vi "CANAnalData.vi"(8 "error in":errorcluster, 9 "ID":u32, 10 "Data":u8[](array[numeric]), 11 "Config":refnum<vi>) -> (0 "error out":errorcluster, 1 "DataLen":u8, 2 "Data out":u8[](array[numeric]), 3 "ID out":u32, 5 "TimeStamp":u32)   [LabVIEW 2017]
uses:
  PCAN_Driver/ControlCAN.llb/VCI_CAN_OBJ.ctl
  Marvin ATP Remake 6.5.18 - Copy/PCAN_Driver/ControlCAN.lvlib
panel:
  in  "cnd_in":u32
  out "cnt_out":u32
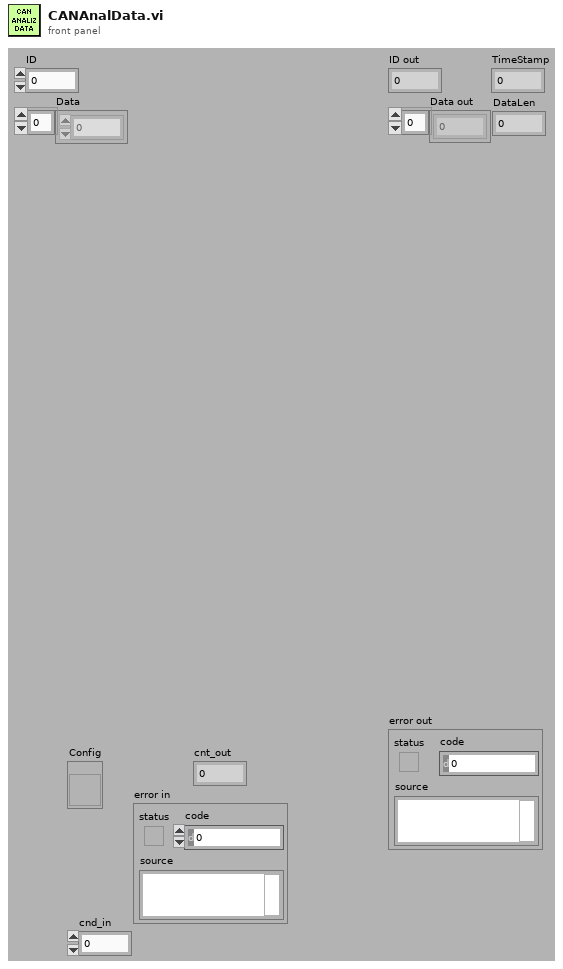
[diagram p1: front panel]
types:
  T1 = typedef "ControlCAN.lvlib/VCI_CAN_OBJ.ctl" = cluster{"ID":u32, "TimeStamp":u32, "TimeFlag":u8, "SendType":u8, "RemoteFlag":u8, "ExternFlag":u8, "DataLen":u8, "Data":u8[], "Reserved":u8[]}
  T2 = typedef "ControlCAN.lvlib/DevType.ctl" = u32
  T3 = typedef "ControlCAN.lvlib/CAN Channel.ctl" = u32
  T4 = typedef "ControlCAN.lvlib/VCI_INIT_CONFIG.ctl" = cluster{"AccCode":u32, "AccMask":u32, "InitFlag":T5, "Fliter":T6, "Timing0":u8, "Timing1":u8, "Mode":T7}
  T5 = typedef "ControlCAN.lvlib/InitFlag.ctl" = u32
  T6 = typedef "ControlCAN.lvlib/Fliter.ctl" = u8
  T7 = typedef "ControlCAN.lvlib/Mode.ctl" = u8
  T8 = cluster{"DevType":T2, "DevIndex":u32, "CanIndex":T3, "VCI_INIT_CONFIG":T4}
  T9 = cluster{"Type":enum16{"接收", "发送"}, "Channel":T3, "Time":timestamp, "VCI_CAN_OBJ":T1}[]
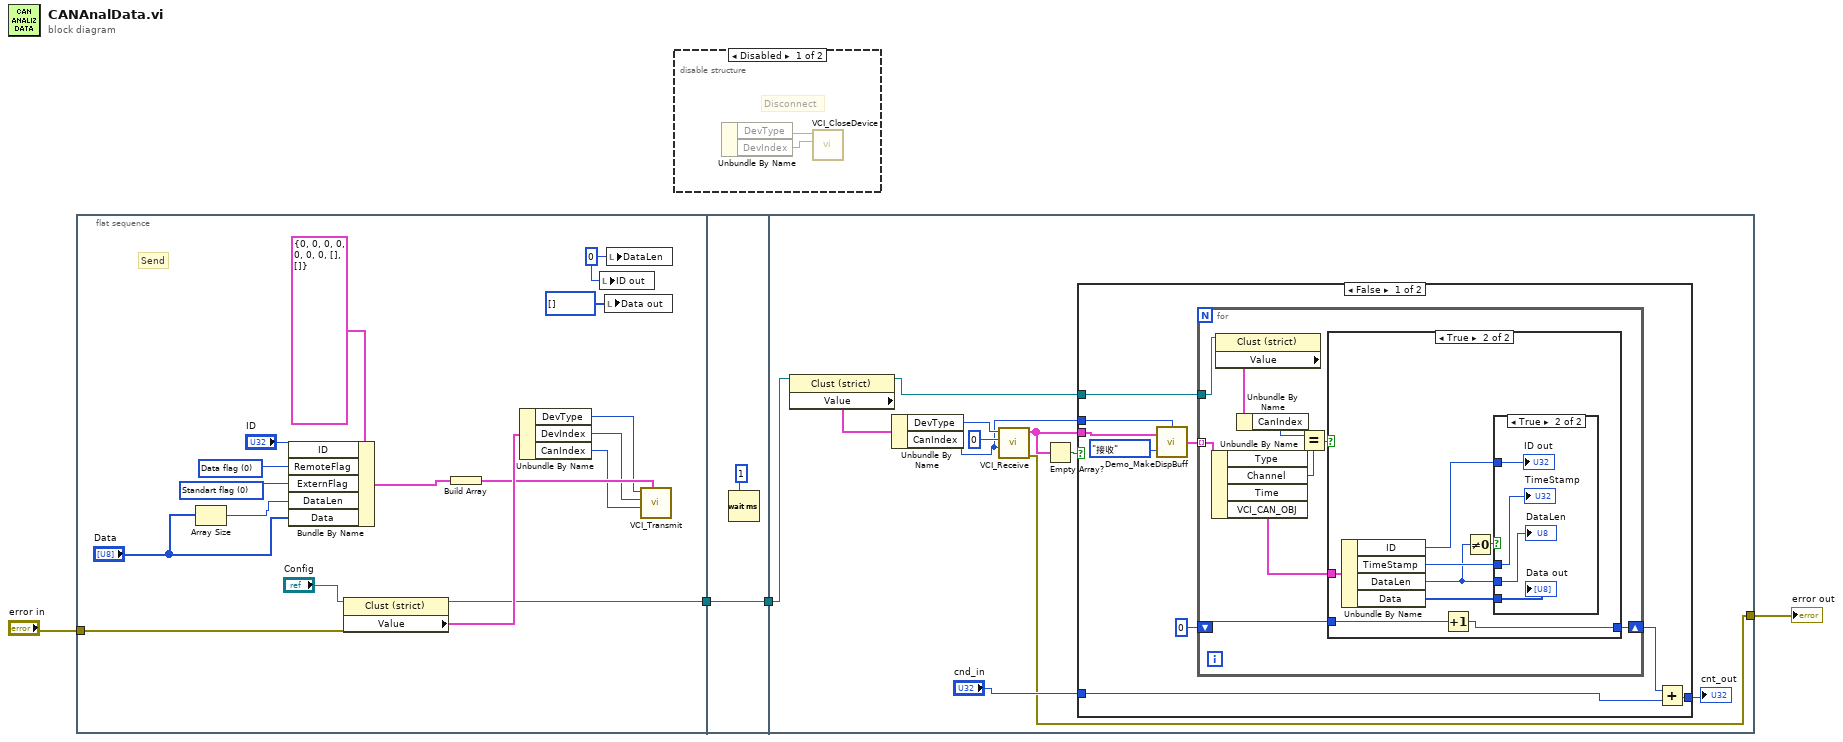
[diagram p0: block diagram]
diagram:
  n1 = flat-sequence {
    tunnel: [w8] -> w4
    tunnel: "error in" -> [w5]
    tunnel: w4 -> [w23]
    tunnel: [w23] -> w3
    tunnel: w3 -> [w25]
    tunnel: [w24] -> w1
    frame #0 {
      w7 = u8 0 ("DataLen")
      w15 = u8 0 items=["Standart flag", "Extern flag"] ("Format")
      w14 = u8 0 items=["Data flag", "Remote flag"] ("Type")
      # "Send"
      n2 = Array Size(array="Data") -> (size(s)=w10:i32)
      n3 = Bundle By Name(cluster=T1 {"ID"=0, "TimeStamp"=0, "TimeFlag"=0, "SendType"=0, "RemoteFlag"=0, "ExternFlag"=0, "DataLen"=0, "Data"=[], "Reserved"=[]} ("Send"), "ID"="ID", "RemoteFlag"=w14, "ExternFlag"=w15, "DataLen"=w10, "Data"="Data") -> (w13:T1)
      n4 = property class="Clust (strict)"(reference="Config", error in=w5) -> (reference out=w8:refnum<vi>, "Value"=w21:T8)  [unwired: 1 out]
      n5 = Build Array(w13) -> (w20:T1[])
      n6 = Unbundle By Name(w21) -> ("DevType"=w17:T2, "DevIndex"=w18:u32, "CanIndex"=w19:T3)
      n7 = local write "ID out"(w7) -> ()
      n8 = local write "Data out"(u8[] [] ("Data out")) -> ()
      n9 = local write "DataLen"(w7) -> ()
      n10 = call "VCI_Transmit.vi"("Buffer"=w20, "CANIndex"=w19, "DevIndex"=w18, "DevType"=w17) -> ()  [unwired: 1 in, 7 out]
    }
    frame #1 {
      n11 = Wait (ms)(milliseconds to wait=u32 1) -> ()  [unwired: 1 out]
    }
    frame #2 {
      n12 = property class="Clust (strict)"(reference=w25) -> (reference out=w34:refnum<vi>, "Value"=w28:T8)  [unwired: 1 in, 1 out]
      n13 = Unbundle By Name(w28) -> ("DevType"=w30:T2, "CanIndex"=w29:T3)
      n14 = call "VCI_Receive.vi"("CANIndex"=w29, "DevIndex"=u32 0, "DevType"=w30) -> ("error out"=w24:errorcluster, "Recieve"=w31:T1[])  [unwired: 3 in, 4 out]
      n15 = Empty Array?(array=w31) -> (empty?=w32:bool)
      n16 = case shown="False" w32 {
        tunnel: w31 -> [w41 _]
        tunnel: w29 -> [w42 _]
        tunnel: "cnd_in" -> [w37 w66]
        tunnel: [w36 w66] -> w27
        tunnel: w34 -> [w35 _]
        frame False {
          n17 = call "Demo_MakeDispBuff.vi"("Channel"=w42, "Type"=enum16{"接收", "发送"}."接收", "OBJs"=w41) -> ("Buffer"=w40:T9)
          n18 = for {
            tunnel: w40 -> [w52] mode=indexing
            shift-right: [w45] -> w38
            shift-left: u32 0 -> [w46]
            tunnel: w35 -> [w44]
            n19 = Unbundle By Name(w52) -> ("Channel"=w48:T3, "VCI_CAN_OBJ"=w51:T1)  [unwired: 2 out]
            n20 = property class="Clust (strict)"(reference=w44) -> ("Value"=w50:T8)  [unwired: 1 in, 2 out]
            n21 = Unbundle By Name(w50) -> ("CanIndex"=w49:T3)
            n22 = Equal?(x=w49, y=w48) -> (x = y?=w47:bool)
            n23 = case shown="True" w47 {
              tunnel: w51 -> [_ w61]
              tunnel: w46 -> [w53 w60]
              tunnel: [w53 w59] -> w45
              frame False {
              }
              frame True {
                n24 = Unbundle By Name(w61) -> ("ID"=w58:u32, "TimeStamp"=w56:u32, "DataLen"=w55:u8, "Data"=w57:u8[])
                n25 = Increment(x=w60) -> (x+1=w59:u32)
                n26 = Not Equal To 0?(x=w55) -> (x != 0?=w54:bool)
                n27 = case shown="True" w54 {
                  tunnel: w58 -> [_ w65]
                  tunnel: w57 -> [_ w64]
                  tunnel: w56 -> [_ w63]
                  tunnel: w55 -> [_ w62]
                  frame False {
                  }
                  frame True {
                    "ID out" <- w65
                    "Data out" <- w64
                    "TimeStamp" <- w63
                    "DataLen" <- w62
                  }
                }
              }
            }
          }
          n28 = Add(x=w38, y=w37) -> (x+y=w36:u32)
        }
        frame True {
        }
      }
      "cnt_out" <- w27
    }
  }
  n29 = disable-structure shown="Disabled" {
    frame Disabled {
      # "Disconnect"
      n30 = Unbundle By Name() -> ("DevType"=w68:T2, "DevIndex"=w67:u32)  [unwired: 1 in]
      n31 = call "VCI_CloseDevice.vi"("DevIndex"=w67, "DevType"=w68) -> ()  [unwired: 1 in, 9 out]
    }
    frame Enabled {
    }
  }
  "error out" <- w1
